vi "AImotive UDP Sender.vi"(8 "error in (no error)":errorcluster, 10 "stop":bool, 11 "destination address":string="255.255.255.255") -> (0 "error out":errorcluster)   [LabVIEW 2019]
doc: "The UDP protocol differs from TCP in that there is no error-checking with the packets of information that are sent, and thus no guarantee whatsoever that an intended recipient will actually receive a given piece of data.\n\nUDP does offer the ability to \"broadcast\" data across a network--simply specify an IP Address of all ones (255.255.255.255) to attempt to broadcast information network-wide. Keep in mind that routers and other network hardware will generally refuse to forward the broadcast beyond certain points, so the extent of the broadcast will in practice be limited."
panel:
  in  "remote port":u16=61557
  in  "port":u16=61556
  out "current value":dbl
  # "Overview: Sends UDP data to the destination addresses. Set destination address to the server address or to 255.255.255.255 to send to the entire network.\n\nInstructions:\n1. Run the VI and click Start Test\n2. Open Simple UDP - Receiver.vi and follow the instructions on its front panel.\n3. Click Stop to stop the VI."
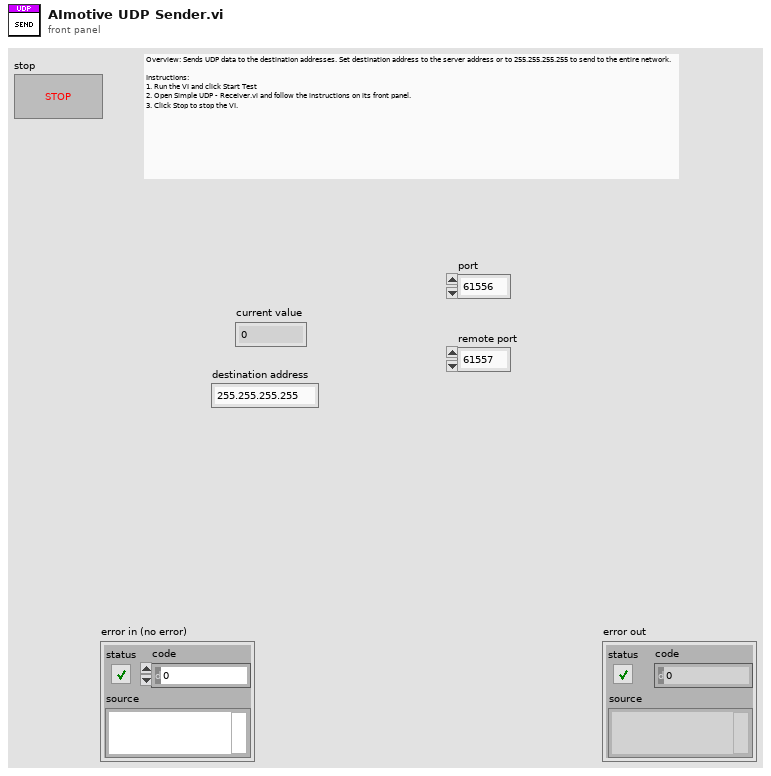
[diagram p1: front panel]
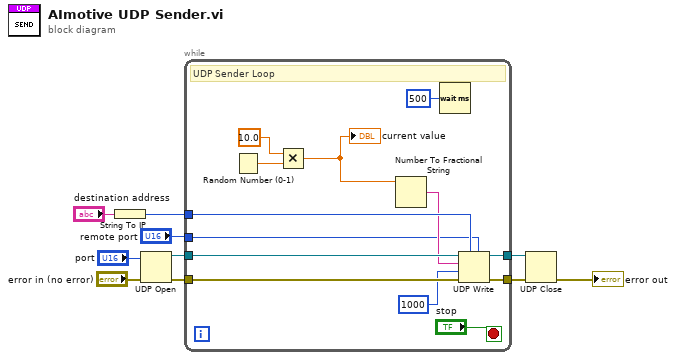
[diagram p0: block diagram]
diagram:
  n1 = String To IP(1:"destination address") -> (0:w5:u32)
  n2 = UDP Open(8:"error in (no error)", 11:"port") -> (port=w4:refnum<k16>, 0:w3:errorcluster)  [unwired: 3 in, 1 out]
  n3 = while {
    tunnel: [w17] -> w7
    tunnel: w4 -> [w23]
    tunnel: w3 -> [w22]
    tunnel: [w21] -> w8
    tunnel: w5 -> [w20]
    tunnel: "remote port" -> [w15]
    stop <- "stop" stop-if-true
    # "UDP Sender Loop"
    n4 = Random Number (0-1)() -> (number: 0 to 1=w13:dbl)
    n5 = Multiply(x=10.0, y=w13) -> (x*y=w11:dbl)
    "current value" <- w11
    n6 = Number To Fractional String(number=w11) -> (F-format string=w18:string)  [unwired: 3 in]
    n7 = Wait (ms)(milliseconds to wait=u32 500) -> ()  [unwired: 1 out]
    n8 = UDP Write(address=w20, port or service name=w15, connection ID=w23, data in=w18, 8:w22, 9:1000 ("timeout ms (25000)")) -> (error out=w17:errorcluster, 3:w21:refnum<k16>)
  }
  n9 = UDP Close(connection ID=w8, 8:w7) -> (error out=→"error out":errorcluster)  [unwired: 1 out]
